vi "lab session 4.vi"() -> ()   [LabVIEW 2020]
uses:
  <vilib>/numeric/Random Number (Range) U64.vi
  <vilib>/numeric/sub_Random U32.vi
panel:
  out "Numeric 2":dbl
  in  "stop":bool
  out "Numeric":i32
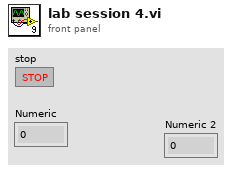
[diagram p1: front panel]
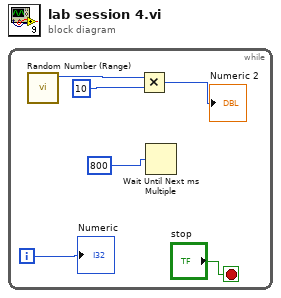
[diagram p0: block diagram]
diagram:
  n1 = while {
    i -> [w6]
    stop <- "stop" stop-if-true
    n2 = call-poly <vilib>:"Random Number (Range).vi"() -> ("number"=w5:u64)  [unwired: 11 in]
    n3 = Multiply(x=w5, y=10) -> (x*y=→"Numeric 2":u64)
    n4 = Wait Until Next ms Multiple(millisecond multiple=800) -> ()  [unwired: 1 out]
    "Numeric" <- w6
  }
